vi "Get Dynamic Methods from Index.vi"(8 "error in (no error)":errorcluster, 10 "Test Case Class Path":path, 11 "Indexing Test Finder in":refnum<class "Indexing Test Finder.lvclass">) -> (0 "error out":errorcluster, 2 "Test Methods":map{string, path}(c390), 3 "Indexing Test Finder out":refnum<class "Indexing Test Finder.lvclass">)   [LabVIEW 2020, in "Indexing Test Finder.lvclass"]
uses:
  Indexing Test Finder.lvclass
  Indexing Test Finder.lvclass/Indexing Test Finder.ctl
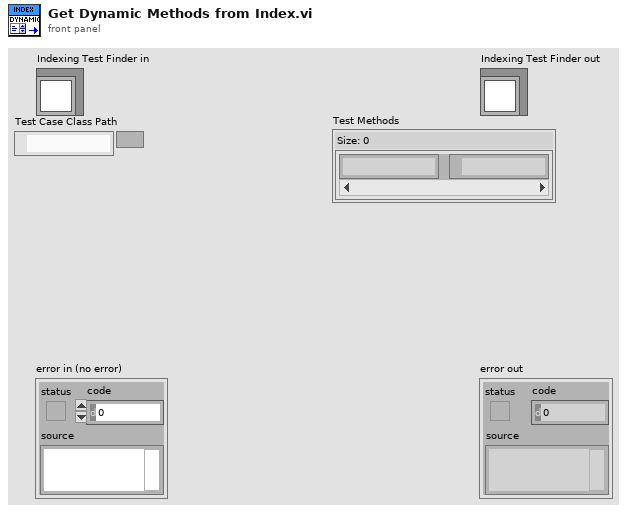
[diagram p1: front panel]
types:
  T1 = typedef "Indexing Test Finder.lvclass/Index Item.ctl" = cluster{"Dynamic Methods":map{string, path}, "Static Methods":map{string, path}, "Signature":string}
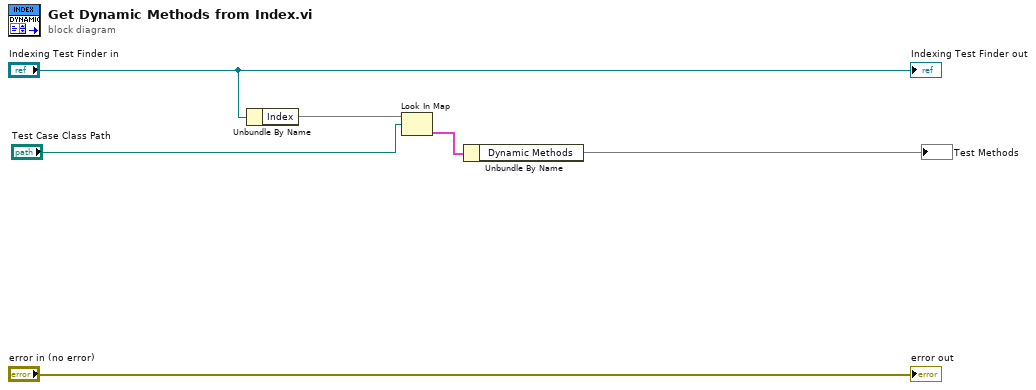
[diagram p0: block diagram]
diagram:
  n1 = Unbundle By Name("Indexing Test Finder in") -> ("Index"=w4:map{path, T1})
  n2 = Look In Map(map=w4, key="Test Case Class Path") -> (value=w2:T1)  [unwired: 1 in, 1 out]
  n3 = Unbundle By Name(w2) -> ("Dynamic Methods"=→"Test Methods":map{string, path})
  "error out" <- "error in (no error)"
  "Indexing Test Finder out" <- "Indexing Test Finder in"
